vi "Set Variant Property.vi"(8 "error in (no error)":errorcluster, 10 "Property In":variant, 11 "2D Compass.lvclass":refnum<class "2D Compass.lvclass">) -> (0 "error out":errorcluster, 3 "2D Compass.lvclass":refnum<class "2D Compass.lvclass">)   [LabVIEW 2017, in "2D Compass.lvclass"]
uses:
  <vilib>/Math Plots/2D Math Plots/2D Compass/2D Compass/2D Compass.lvclass
  <vilib>/Math Plots/2D Math Plots/2D Compass/2D Compass/Typedef/2D Compass Property Cluster.ctl
  <vilib>/Math Plots/2D Math Plots/2D Plot/2D Plot/Typedef/Plot Property Array.ctl
  <vilib>/Math Plots/2D Math Plots/2D Plot/2D Plot/Typedef/Plot Property.ctl
  <vilib>/Math Plots/2D Math Plots/2D Compass/2D Compass/Typedef/2D Compass Property Array.ctl
  <vilib>/Math Plots/2D Math Plots/2D Compass/2D Compass/Typedef/2D Compass Property.ctl
  <vilib>/Math Plots/2D Math Plots/2D Compass/2D Compass/2D Compass.lvclass/2D Compass.ctl
  <vilib>/Math Plots/2D Math Plots/2D Plot/2D Plot/2D Plot.lvclass
panel:
  in  "Compass Property Cluster":T1={"Plot Property Array"=[{"Bar Plot Style"=0, "DigitalLineStyle"=1, "TransitionLocation"=2, "Transition Type"=0, "Fill To"=-1, "Fill/Pt. Color"=16448250, "Label Style"=3, "Line Style"=0, "Line Width"=0, "Plot Color"=16448250, "Plot Interpolation"=0, "Plot Name"="Plot 0", "Point Style"=1, "Visible?"=TRUE, "XScaleIdx"=0, "YScaleIdx"=0}, {"Bar Plot Style"=0, "DigitalLineStyle"=1, "TransitionLocation"=2, "Transition Type"=0, "Fill To"=-1, "Fill/Pt. Color"=16448250, "Label Style"=3, "Line Style"=0, "Line Width"=0, "Plot Color"=16448250, "Plot Interpolation"=0, "Plot Name"="Plot 1", "Point Style"=1, "Visible?"=TRUE, "XScaleIdx"=0, "YScaleIdx"=0}], "2D Compass Array"=[{"Compass Size"=2.0}, {"Compass Size"=2.0}], "Scale Visibility"={"Phase Scale"=TRUE}}
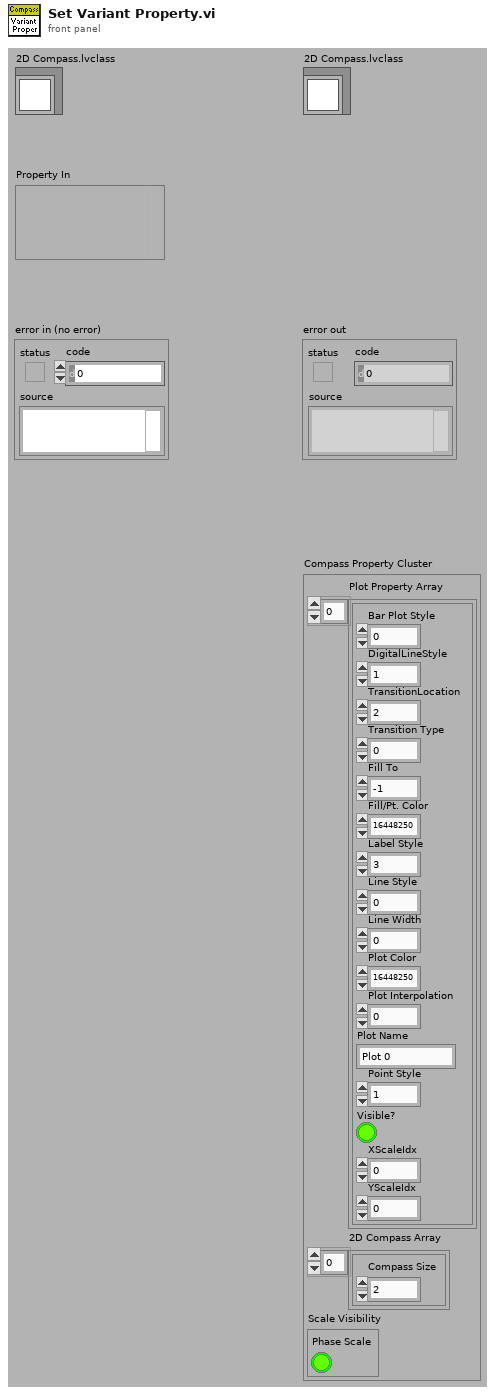
[diagram p1: front panel]
types:
  T1 = typedef "2D Compass.lvclass/2D Compass Property Cluster.ctl" = cluster{"Plot Property Array":T2, "2D Compass Array":T4, "Scale Visibility":cluster{"Phase Scale":bool}}
  T2 = typedef "2D Plot.lvclass/Plot Property Array.ctl" = T3[]
  T3 = typedef "2D Plot.lvclass/Plot Property.ctl" = cluster{"Bar Plot Style":u8, "DigitalLineStyle":u8, "TransitionLocation":u8, "Transition Type":u8, "Fill To":i16, "Fill/Pt. Color":u32, "Label Style":u8, "Line Style":u8, "Line Width":u8, "Plot Color":u32, "Plot Interpolation":u8, "Plot Name":string, "Point Style":u8, "Visible?":bool, "XScaleIdx":u32, "YScaleIdx":u32}
  T4 = typedef "2D Compass.lvclass/2D Compass Property Array.ctl" = T5[]
  T5 = typedef "2D Compass.lvclass/2D Compass Property.ctl" = cluster{"Compass Size":dbl}
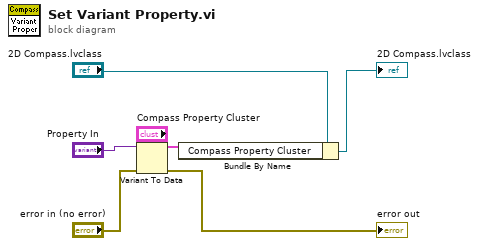
[diagram p0: block diagram]
diagram:
  n1 = Variant To Data(error in="error in (no error)", type="Compass Property Cluster", Variant="Property In") -> (data=w7:T1, error out=→"error out":errorcluster)
  n2 = Bundle By Name(cluster="2D Compass.lvclass", "Compass Property Cluster"=w7) -> (→"2D Compass.lvclass":refnum<class "2D Compass.lvclass">)
